vi "GFITS_SetTestVars.vi"(9 "testbname":string="test", 10 "testdir":path=path "/tmp", 11 "Database RefNum in":T1) -> ()   [LabVIEW 2016]
uses:
  DBSHAND/private/vis/DatabaseHand_RefNum.ctl
  DBSHAND/private/vis/DatabaseHand_Element_Set(path).vi
  DBSHAND/private/vis/DatabaseHand_Element_Set(string).vi
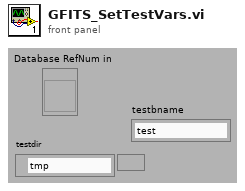
[diagram p1: front panel]
types:
  T1 = typedef "DatabaseHand_RefNum.ctl" = refnum<vi>
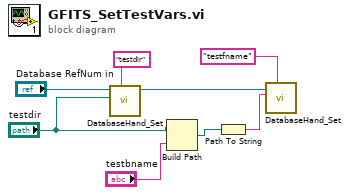
[diagram p0: block diagram]
diagram:
  n1 = call-poly "DatabaseHand_Set.vi"("name"="testdir", "value"="testdir", "Database RefNum in"="Database RefNum in") -> ("Database RefNum out"=w2:T1)  [unwired: 5 in, 3 out]
  n2 = Build Path(base path="testdir", name or relative path="testbname") -> (appended path=w4:path)
  n3 = Path To String(path=w4) -> (string=w3:string)
  n4 = call-poly "DatabaseHand_Set.vi"("name"="testfname", "value"=w3, "Database RefNum in"=w2) -> ()  [unwired: 5 in, 4 out]
